vi "pov to bool(Hold).vi"(11 "Numeric":i16) -> (0 "Left":bool, 1 "Down":bool, 2 "Up":bool, 3 "Right":bool)   [LabVIEW 2019, in "Joysticks.lvlib" / "Joysticks.lvclass"]
doc: "This VI takes the D-Pad actions into 4 seperate outputs."
uses:
  Joysticks.lvclass
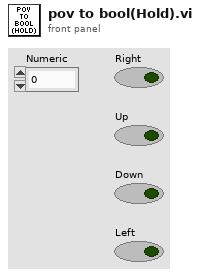
[diagram p1: front panel]
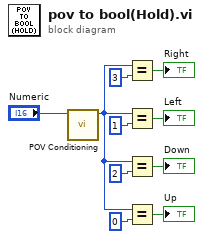
[diagram p0: block diagram]
diagram:
  n1 = call "POV Conditioning.vi"("POV"="Numeric") -> ("Output [-1-4]"=w9:i16)  [unwired: 10 in]
  n2 = Equal?(x=w9, y=i16 3) -> (x = y?=→"Right":bool)
  n3 = Equal?(x=w9, y=i16 1) -> (x = y?=→"Left":bool)
  n4 = Equal?(x=w9, y=i16 2) -> (x = y?=→"Down":bool)
  n5 = Equal?(x=w9, y=i16 0) -> (x = y?=→"Up":bool)
